vi "Read Actual Voltage Array.vi"(8 "error in (no error)":errorcluster, 11 "Mode in":refnum<class "Mode.lvclass">) -> (0 "error out":errorcluster, 2 "Actual Voltage Array":dbl[](array[numeric]), 3 "Mode out":refnum<class "Mode.lvclass">)   [LabVIEW 2019, in "Mode.lvclass"]
uses:
  Mode.lvclass
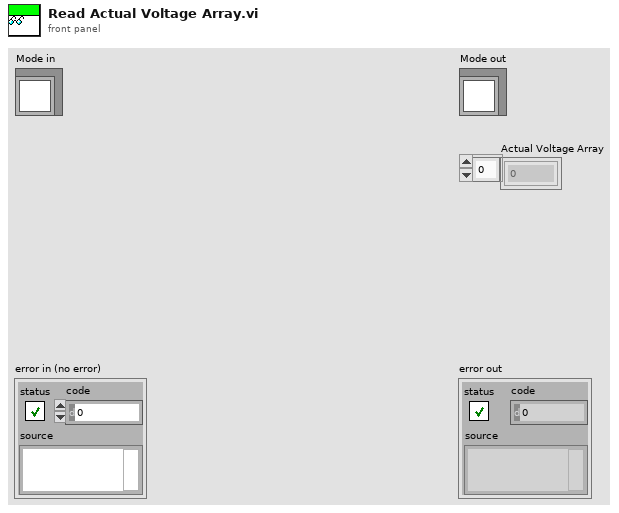
[diagram p1: front panel]
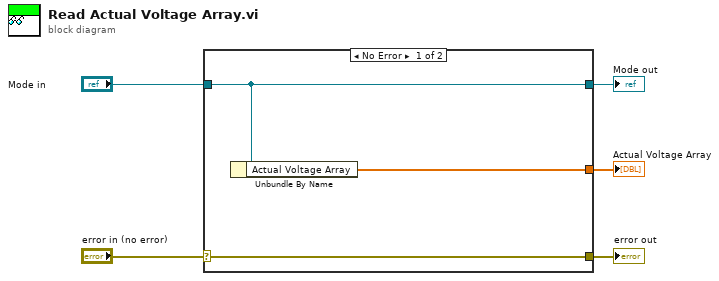
[diagram p0: block diagram]
diagram:
  n1 = case shown="No Error" "error in (no error)" {
    selector: "error in (no error)" -> [w8 w9]
    tunnel: [w8 w9] -> w4
    tunnel: [w7 w10] -> w2
    tunnel: "Mode in" -> [w7 w10]
    tunnel: [w6 _] -> w1
    frame No Error {
      n2 = Unbundle By Name(w7) -> ("Actual Voltage Array"=w6:dbl[])
    }
    frame Error {
    }
  }
  "error out" <- w4
  "Mode out" <- w2
  "Actual Voltage Array" <- w1
